vi "Speed Transformation with Acceleration and Actual Speed FeedBack 18.06.19.vi"(3 "wTargetSpeed":dbl, 4 "yTargetSpeed":dbl, 5 "xTargetSpeed":dbl) -> (0 "Output Distance":T1, 2 "Output\nSpeed":T2)   [LabVIEW 2018]
panel:
  in  "Boolean":bool=TRUE
  out "Time Elapsed":dbl
  out "current time":timestamp
  out "Time Start":timestamp
  out "Waveform Chart 3":dbl(graph)
  out "Waveform Chart 2":dbl(graph)
  out "Waveform Chart":dbl(graph)
  out "Distance & Speed Cluster":T3
  in  "stop":bool
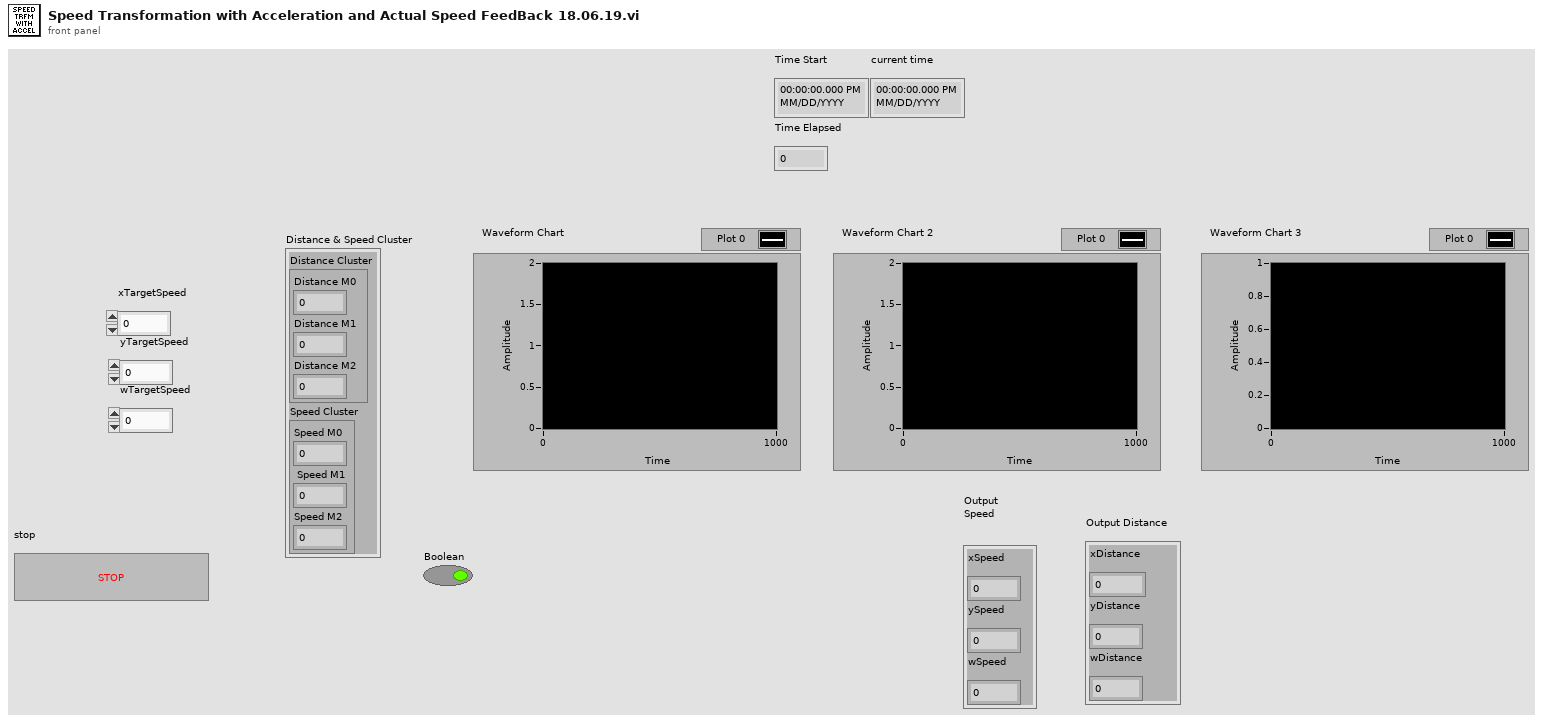
[diagram p1: front panel]
types:
  T1 = cluster{"xDistance":dbl, "yDistance":dbl, "wDistance":dbl}
  T2 = cluster{"xSpeed":dbl, "ySpeed":dbl, "wSpeed":dbl}
  T3 = cluster{"Distance Cluster":cluster{"Distance M0 ":dbl, "Distance M1 ":dbl, "Distance M2 ":dbl}, "Speed Cluster":cluster{"Speed M0":dbl, " Speed M1":dbl, "Speed M2":dbl}}
  T4 = cluster{"Distance M0 ":dbl, "Distance M1 ":dbl, "Distance M2 ":dbl}
  T5 = cluster{"Speed M0":dbl, " Speed M1":dbl, "Speed M2":dbl}
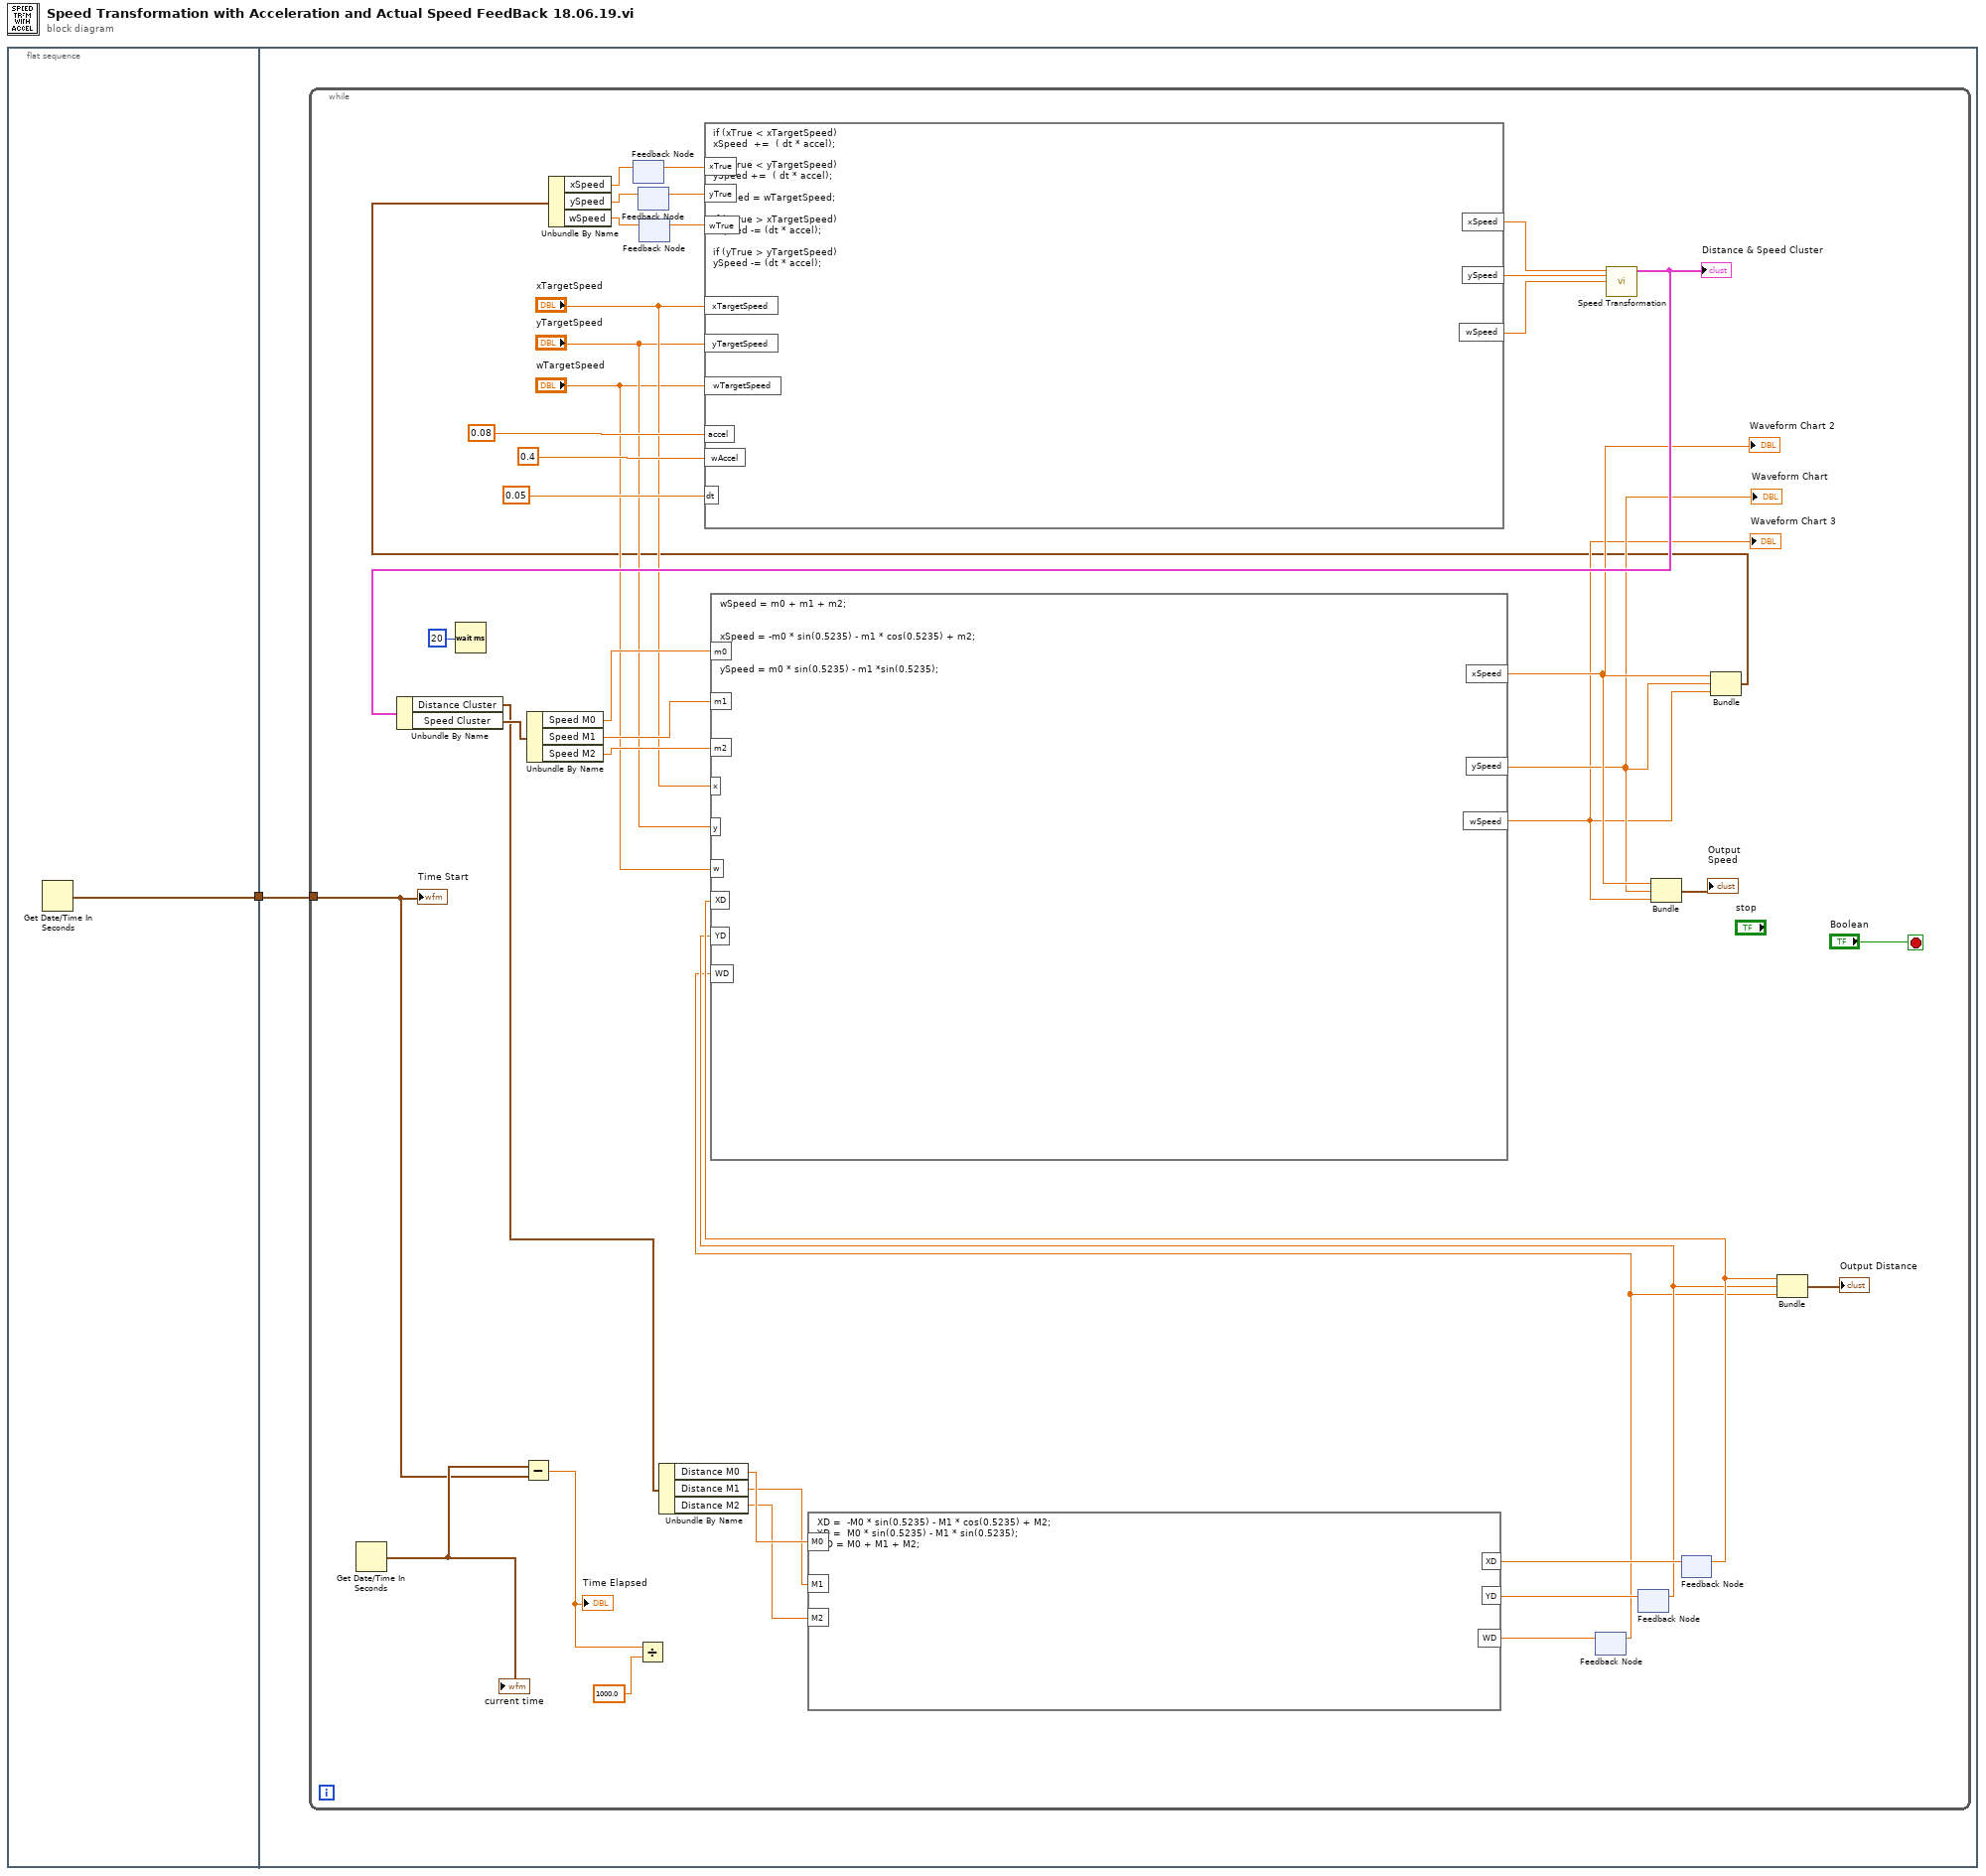
[diagram p0: block diagram]
diagram:
  n1 = flat-sequence {
    tunnel: [w2] -> w1
    tunnel: w1 -> [w3]
    frame #0 {
      n2 = Get Date/Time In Seconds() -> (seconds since 1Jan1904=w2:timestamp)
    }
    frame #1 {
      n3 = while {
        tunnel: w3 -> [w29]
        stop <- "Boolean" stop-if-true
        n4 = Get Date/Time In Seconds() -> (seconds since 1Jan1904=w30:timestamp)
        "current time" <- w30
        n5 = Wait (ms)(milliseconds to wait=u32 20) -> ()  [unwired: 1 out]
        n6 = Subtract(x=w30, y=w29) -> (x-y=w28:dbl)
        "Time Elapsed" <- w28
        n7 = feedback #1() -> (w9:dbl)  [unwired: 1 in]
        n8 = Divide(x=w28, y=1000.0) -> ()  [unwired: 1 out]
        n9 = feedback #2() -> (w7:dbl)  [unwired: 1 in]
        n10 = feedback #3() -> (w5:dbl)  [unwired: 1 in]
        n11 = formula code="if (xTrue < xTargetSpeed)\nxSpeed  +=  ( dt * accel);\n\nif (yTrue < yTargetSpeed)\nySpeed +=  ( dt * accel);\n\nwSpeed = wTargetSpeed;\n\nif (xTrue > xTargetSpeed)\nxSpeed -= (dt * accel);\n\nif (yTrue > yTargetSpeed)\nySpeed -= (dt * accel);"("xTargetSpeed"="xTargetSpeed", "yTargetSpeed"="yTargetSpeed", "wTargetSpeed"="wTargetSpeed", "accel"=0.08 ("input variable"), "dt"=0.05 ("input variable"), "wAccel"=0.4 ("input variable"), "xTrue"=w9, "yTrue"=w7, "wTrue"=w5) -> ("xSpeed"=w45:dbl, "ySpeed"=w44:dbl, "wSpeed"=w43:dbl)
        n12 = feedback #4() -> (w15:dbl)  [unwired: 1 in]
        n13 = call "Speed Transformation.vi"("w"=w43, "Vy"=w44, "Vx"=w45) -> ("Distance & Speed Cluster"=w34:T3)  [unwired: 8 in]
        "Distance & Speed Cluster" <- w34
        n14 = Unbundle By Name(w34) -> ("Distance Cluster"=w21:T4, "Speed Cluster"=w38:T5)
        n15 = Unbundle By Name(w38) -> ("Speed M0"=w37:dbl, "Speed M1"=w36:dbl, "Speed M2"=w35:dbl)
        n16 = Unbundle By Name(w21) -> ("Distance M0"=w20:dbl, "Distance M1"=w19:dbl, "Distance M2"=w18:dbl)
        n17 = formula code="XD =  -M0 * sin(0.5235) - M1 * cos(0.5235) + M2; \nYD =  M0 * sin(0.5235) - M1 * sin(0.5235);\nWD = M0 + M1 + M2;"("M0"=w20, "M1"=w19, "M2"=w18) -> ("XD"=w26:dbl, "YD"=w25:dbl, "WD"=w24:dbl)
        n18 = feedback-in #4(w24) -> ()
        n19 = feedback-in #5(w25) -> ()
        n20 = feedback #5() -> (w16:dbl)  [unwired: 1 in]
        n21 = feedback-in #6(w26) -> ()
        n22 = feedback #6() -> (w17:dbl)  [unwired: 1 in]
        n23 = formula code="wSpeed = m0 + m1 + m2;\n\n\nxSpeed = -m0 * sin(0.5235) - m1 * cos(0.5235) + m2;\n\n\nySpeed = m0 * sin(0.5235) - m1 *sin(0.5235);"("m0"=w37, "m1"=w36, "m2"=w35, "x"="xTargetSpeed", "y"="yTargetSpeed", "w"="wTargetSpeed", "XD"=w17, "YD"=w16, "WD"=w15) -> ("ySpeed"=w13:dbl, "xSpeed"=w14:dbl, "wSpeed"=w12:dbl)
        "Waveform Chart" <- w13
        "Waveform Chart 2" <- w14
        "Waveform Chart 3" <- w12
        n24 = Bundle("xSpeed"=w14, "ySpeed"=w13, "wSpeed"=w12) -> (→"Output\nSpeed":T2)  [unwired: 1 in]
        n25 = Bundle("xSpeed"=w14, "ySpeed"=w13, "wSpeed"=w12) -> (w11:T2)  [unwired: 1 in]
        n26 = Unbundle By Name(w11) -> ("xSpeed"=w10:dbl, "ySpeed"=w8:dbl, "wSpeed"=w6:dbl)
        n27 = feedback-in #1(w10) -> ()
        n28 = feedback-in #2(w8) -> ()
        n29 = feedback-in #3(w6) -> ()
        n30 = Bundle("XD"=w17, "YD"=w16, "WD"=w15) -> (→"Output Distance":cluster{"XD":dbl, "YD":dbl, "WD":dbl})  [unwired: 1 in]
        "Time Start" <- w29
      }
    }
  }
